vi "Set Bucket Request Payment.vi"(8 "error in (no error)":errorcluster, 10 "Payer":T1, 11 "Bucket in":refnum<class "Bucket.lvclass">) -> (0 "error out":errorcluster, 3 "Bucket out":refnum<class "Bucket.lvclass">)   [LabVIEW 2015, in "NI_AWS_S3.lvlib" / "Bucket.lvclass"]
doc: "This implementation of the PUT operation uses the requestPayment subresource to set the request payment configuration of a bucket. By default, the bucket owner pays for downloads from the bucket. This configuration parameter enables the bucket owner (only) to specify that the person requesting the download will be charged for the download."
uses:
  Bucket.lvclass
  Payer.ctl
  Core/HTTP Request/Region handling.ctl
  Core/HTTP Request/Request Options.ctl
  Core/HTTP Request/Name Value Pair.ctl
  Core/HTTP Request/URL formatting.ctl
  Bucket.lvclass/Bucket.ctl
  Read Name.vi
  Core/HTTP Request/HTTP Request.lvclass
  NI_AWS_S3.lvlib
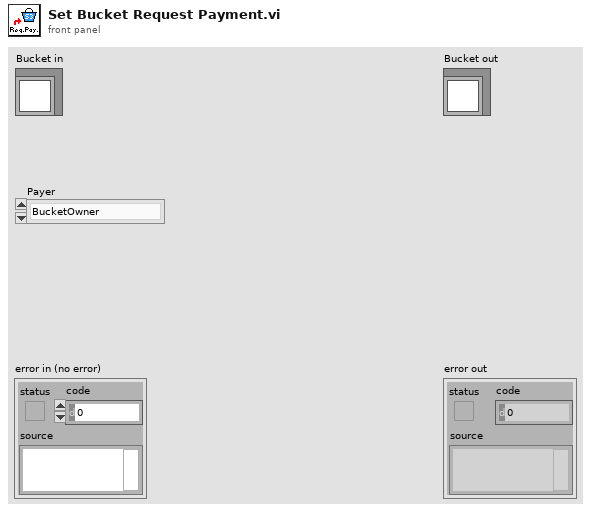
[diagram p1: front panel]
types:
  T1 = typedef "NI_AWS_S3.lvlib/Payer.ctl" = enum16{"BucketOwner", "Requester"}
  T2 = typedef "NI_AWS_Core.lvlib/HTTP Request.lvclass/Name Value Pair.ctl" = cluster{"name":string, "value":string}
  T3 = typedef "NI_AWS_Core.lvlib/HTTP Request.lvclass/Request Options.ctl" = cluster{"request headers":T2[], "request parameters":T2[], "request body":string, "region handling":T4, "URL formatting":T5}
  T4 = typedef "NI_AWS_Core.lvlib/HTTP Request.lvclass/Region handling.ctl" = enum16{"use region everywhere", "use region (authentication only)", "use region (URL only)", "ignore region everwhere"}
  T5 = typedef "NI_AWS_Core.lvlib/HTTP Request.lvclass/URL formatting.ctl" = enum16{"region-", "region."}
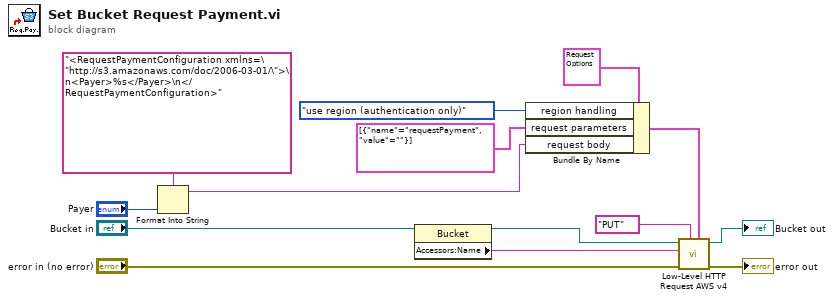
[diagram p0: block diagram]
diagram:
  n1 = Format Into String(format string="<RequestPaymentConfiguration xmlns=\"http://s3.amazonaws.com/doc/2006-03-01/\">\n<Payer>%s</Payer>\n</RequestPaymentConfiguration>", "Payer") -> (resulting string=w1:string)  [unwired: 2 in, 1 out]
  n2 = property class="Bucket"(reference="Bucket in") -> (reference out=w5:refnum<class "Bucket.lvclass">, "Accessors:Name"=w14:string)  [unwired: 1 in, 1 out]
  n3 = Bundle By Name(cluster=T3 {"request headers"=[], "request parameters"=[], "request body"="", "region handling"=enum."use region everywhere", "URL formatting"=enum."region."} ("Request Options"), "region handling"=Region_handling."use region (authentication only)", "request parameters"=T2[] [{"name"="requestPayment", "value"=""}], "request body"=w1) -> (w6:T3)
  n4 = call "Low-Level HTTP Request AWS v4.vi"("Request Options"=w6, "HTTP-Verb"="PUT", "error in (no error)"="error in (no error)", "URL Prefix"=w14, "AWS Core in"=w5) -> ("error out"=→"error out":errorcluster, "AWS Core out"=→"Bucket out":refnum<class "Bucket.lvclass">)  [unwired: 3 in, 2 out]
